vi "test TCX read (installed 71).vi"() -> ()   [LabVIEW 2011] (continued)
2\"><Watts>150</Watts></TPX></Extensions></Trackpoint><Trackpoint><Time>2008-03-03T23:14:53Z</Time><Position><LatitudeDegrees>35.869608</LatitudeDegrees><LongitudeDegrees>-78.914474</LongitudeDegrees></Position><AltitudeMeters>67.430</AltitudeMeters><DistanceMeters>16349.594</DistanceMeters><Cadence>80</Cadence><Extensions><TPX xmlns=\"http://www.garmin.com/xmlschemas/ActivityExtension/v2\"><Watts>150</Watts></TPX></Extensions></Trackpoint><Trackpoint><Time>2008-03-03T23:14:54Z</Time><Position><LatitudeDegrees>35.869697</LatitudeDegrees><LongitudeDegrees>-78.914429</LongitudeDegrees></Position><AltitudeMeters>66.949</AltitudeMeters><DistanceMeters>16360.299</DistanceMeters><Cadence>80</Cadence><Extensions><TPX xmlns=\"http://www.garmin.com/xmlschemas/ActivityExtension/v2\"><Watts>127</Watts></TPX></Extensions></Trackpoint><Trackpoint><Time>2008-03-03T23:14:55Z</Time><Position><LatitudeDegrees>35.869785</LatitudeDegrees><LongitudeDegrees>-78.914384</LongitudeDegrees></Position><AltitudeMeters>67.430</AltitudeMeters><DistanceMeters>16370.849</DistanceMeters><Cadence>80</Cadence><Extensions><TPX xmlns=\"http://www.garmin.com/xmlschemas/ActivityExtension/v2\"><Watts>124</Watts></TPX></Extensions></Trackpoint><Trackpoint><Time>2008-03-03T23:14:56Z</Time><Position><LatitudeDegrees>35.869873</LatitudeDegrees><LongitudeDegrees>-78.914337</LongitudeDegrees></Position><AltitudeMeters>67.430</AltitudeMeters><DistanceMeters>16381.465</DistanceMeters><Cadence>80</Cadence><Extensions><TPX xmlns=\"http://www.garmin.com/xmlschemas/ActivityExtension/v2\"><Watts>125</Watts></TPX></Extensions></Trackpoint><Trackpoint><Time>2008-03-03T23:14:57Z</Time><Position><LatitudeDegrees>35.869961</LatitudeDegrees><LongitudeDegrees>-78.914292</LongitudeDegrees></Position><AltitudeMeters>66.949</AltitudeMeters><DistanceMeters>16392.021</DistanceMeters><Cadence>81</Cadence><Extensions><TPX xmlns=\"http://www.garmin.com/xmlschemas/ActivityExtension/v2\"><Watts>138</Watts></TPX></Extensions></Trackpoint><Trackpoint><Time>2008-03-03T23:14:58Z</Time><Position><LatitudeDegrees>35.870049</LatitudeDegrees><LongitudeDegrees>-78.914246</LongitudeDegrees></Position><AltitudeMeters>66.468</AltitudeMeters><DistanceMeters>16402.668</DistanceMeters><Cadence>81</Cadence><Extensions><TPX xmlns=\"http://www.garmin.com/xmlschemas/ActivityExtension/v2\"><Watts>140</Watts></TPX></Extensions></Trackpoint><Trackpoint><Time>2008-03-03T23:14:59Z</Time><Position><LatitudeDegrees>35.870137</LatitudeDegrees><LongitudeDegrees>-78.914199</LongitudeDegrees></Position><AltitudeMeters>65.988</AltitudeMeters><DistanceMeters>16413.375</DistanceMeters><Cadence>81</Cadence><Extensions><TPX xmlns=\"http://www.garmin.com/xmlschemas/ActivityExtension/v2\"><Watts>126</Watts></TPX></Extensions></Trackpoint><Trackpoint><Time>2008-03-03T23:15:00Z</Time><Position><LatitudeDegrees>35.870228</LatitudeDegrees><LongitudeDegrees>-78.914151</LongitudeDegrees></Position><AltitudeMeters>65.507</AltitudeMeters><DistanceMeters>16424.277</DistanceMeters><Cadence>80</Cadence><Extensions><TPX xmlns=\"http://www.garmin.com/xmlschemas/ActivityExtension/v2\"><Watts>119</Watts></TPX></Extensions></Trackpoint><Trackpoint><Time>2008-03-03T23:15:01Z</Time><Position><LatitudeDegrees>35.870317</LatitudeDegrees><LongitudeDegrees>-78.914102</LongitudeDegrees></Position><AltitudeMeters>65.026</AltitudeMeters><DistanceMeters>16435.098</DistanceMeters><Cadence>78</Cadence><Extensions><TPX xmlns=\"http://www.garmin.com/xmlschemas/ActivityExtension/v2\"><Watts>109</Watts></TPX></Extensions></Trackpoint><Trackpoint><Time>2008-03-03T23:15:02Z</Time><Position><LatitudeDegrees>35.870407</LatitudeDegrees><LongitudeDegrees>-78.914053</LongitudeDegrees></Position><AltitudeMeters>65.026</AltitudeMeters><DistanceMeters>16446.086</DistanceMeters><Cadence>79</Cadence><Extensions><TPX xmlns=\"http://www.garmin.com/xmlschemas/ActivityExtension/v2\"><Watts>111</Watts></TPX></Extensions></Trackpoint><Trackpoint><Time>2008-03-03T23:15:03Z</Time><Position><LatitudeDegrees>35.870499</LatitudeDegrees><LongitudeDegrees>-78.914004</LongitudeDegrees></Position><AltitudeMeters>65.026</AltitudeMeters><DistanceMeters>16457.268</DistanceMeters><Cadence>80</Cadence><Extensions><TPX xmlns=\"http://www.garmin.com/xmlschemas/ActivityExtension/v2\"><Watts>116</Watts></TPX></Extensions></Trackpoint><Trackpoint><Time>2008-03-03T23:15:04Z</Time><Position><LatitudeDegrees>35.870594</LatitudeDegrees><LongitudeDegrees>-78.913954</LongitudeDegrees></Position><AltitudeMeters>64.065</AltitudeMeters><DistanceMeters>16468.787</DistanceMeters><Cadence>82</Cadence><Extensions><TPX xmlns=\"http://www.garmin.com/xmlschemas/ActivityExtension/v2\"><Watts>159</Watts></TPX></Extensions></Trackpoint><Trackpoint><Time>2008-03-03T23:15:05Z</Time><Position><LatitudeDegrees>35.870692</LatitudeDegrees><LongitudeDegrees>-78.913902</LongitudeDegrees></Position><AltitudeMeters>63.584</AltitudeMeters><DistanceMeters>16480.574</DistanceMeters><Cadence>84</Cadence><Extensions><TPX xmlns=\"http://www.garmin.com/xmlschemas/ActivityExtension/v2\"><Watts>189</Watts></TPX></Extensions></Trackpoint><Trackpoint><Time>2008-03-03T23:15:06Z</Time><Position><LatitudeDegrees>35.870793</LatitudeDegrees><LongitudeDegrees>-78.913849</LongitudeDegrees></Position><AltitudeMeters>63.584</AltitudeMeters><DistanceMeters>16492.729</DistanceMeters><Cadence>86</Cadence><Extensions><TPX xmlns=\"http://www.garmin.com/xmlschemas/ActivityExtension/v2\"><Watts>188</Watts></TPX></Extensions></Trackpoint><Trackpoint><Time>2008-03-03T23:15:07Z</Time><Position><LatitudeDegrees>35.870897</LatitudeDegrees><LongitudeDegrees>-78.913795</LongitudeDegrees></Position><AltitudeMeters>63.584</AltitudeMeters><DistanceMeters>16505.369</DistanceMeters><Cadence>88</Cadence><Extensions><TPX xmlns=\"http://www.garmin.com/xmlschemas/ActivityExtension/v2\"><Watts>169</Watts></TPX></Extensions></Trackpoint><Trackpoint><Time>2008-03-03T23:15:08Z</Time><Position><LatitudeDegrees>35.871002</LatitudeDegrees><LongitudeDegrees>-78.913740</LongitudeDegrees></Position><AltitudeMeters>63.104</AltitudeMeters><DistanceMeters>16518.016</DistanceMeters><Cadence>89</Cadence><Extensions><TPX xmlns=\"http://www.garmin.com/xmlschemas/ActivityExtension/v2\"><Watts>127</Watts></TPX></Extensions></Trackpoint><Trackpoint><Time>2008-03-03T23:15:09Z</Time><Position><LatitudeDegrees>35.871109</LatitudeDegrees><LongitudeDegrees>-78.913686</LongitudeDegrees></Position><AltitudeMeters>61.662</AltitudeMeters><DistanceMeters>16530.844</DistanceMeters><Cadence>92</Cadence><Extensions><TPX xmlns=\"http://www.garmin.com/xmlschemas/ActivityExtension/v2\"><Watts>98</Watts></TPX></Extensions></Trackpoint><Trackpoint><Time>2008-03-03T23:15:10Z</Time><Position><LatitudeDegrees>35.871217</LatitudeDegrees><LongitudeDegrees>-78.913629</LongitudeDegrees></Position><AltitudeMeters>62.142</AltitudeMeters><DistanceMeters>16543.873</DistanceMeters><Cadence>93</Cadence><Extensions><TPX xmlns=\"http://www.garmin.com/xmlschemas/ActivityExtension/v2\"><Watts>87</Watts></TPX></Extensions></Trackpoint><Trackpoint><Time>2008-03-03T23:15:11Z</Time><Position><LatitudeDegrees>35.871326</LatitudeDegrees><LongitudeDegrees>-78.913570</LongitudeDegrees></Position><AltitudeMeters>60.700</AltitudeMeters><DistanceMeters>16557.111</DistanceMeters><Cadence>88</Cadence><Extensions><TPX xmlns=\"http://www.garmin.com/xmlschemas/ActivityExtension/v2\"><Watts>91</Watts></TPX></Extensions></Trackpoint><Trackpoint><Time>2008-03-03T23:15:12Z</Time><Position><LatitudeDegrees>35.871438</LatitudeDegrees><LongitudeDegrees>-78.913510</LongitudeDegrees></Position><AltitudeMeters>60.700</AltitudeMeters><DistanceMeters>16570.666</DistanceMeters><Cadence>88</Cadence><Extensions><TPX xmlns=\"http://www.garmin.com/xmlschemas/ActivityExtension/v2\"><Watts>93</Watts></TPX></Extensions></Trackpoint><Trackpoint><Time>2008-03-03T23:15:13Z</Time><Position><LatitudeDegrees>35.871559</LatitudeDegrees><LongitudeDegrees>-78.913447</LongitudeDegrees></Position><AltitudeMeters>61.662</AltitudeMeters><DistanceMeters>16585.230</DistanceMeters><Cadence>90</Cadence><Extensions><TPX xmlns=\"http://www.garmin.com/xmlschemas/ActivityExtension/v2\"><Watts>100</Watts></TPX></Extensions></Trackpoint><Trackpoint><Time>2008-03-03T23:15:14Z</Time><Position><LatitudeDegrees>35.871675</LatitudeDegrees><LongitudeDegrees>-78.913392</LongitudeDegrees></Position><AltitudeMeters>59.739</AltitudeMeters><DistanceMeters>16599.100</DistanceMeters><Cadence>91</Cadence><Extensions><TPX xmlns=\"http://www.garmin.com/xmlschemas/ActivityExtension/v2\"><Watts>165</Watts></TPX></Extensions></Trackpoint><Trackpoint><Time>2008-03-03T23:15:15Z</Time><Position><LatitudeDegrees>35.871797</LatitudeDegrees><LongitudeDegrees>-78.913344</LongitudeDegrees></Position><AltitudeMeters>58.778</AltitudeMeters><DistanceMeters>16613.279</DistanceMeters><Cadence>91</Cadence><Extensions><TPX xmlns=\"http://www.garmin.com/xmlschemas/ActivityExtension/v2\"><Watts>165</Watts></TPX></Extensions></Trackpoint><Trackpoint><Time>2008-03-03T23:15:16Z</Time><Position><LatitudeDegrees>35.871917</LatitudeDegrees><LongitudeDegrees>-78.913298</LongitudeDegrees></Position><AltitudeMeters>58.778</AltitudeMeters><DistanceMeters>16627.301</DistanceMeters><Cadence>91</Cadence><Extensions><TPX xmlns=\"http://www.garmin.com/xmlschemas/ActivityExtension/v2\"><Watts>150</Watts></TPX></Extensions></Trackpoint><Trackpoint><Time>2008-03-03T23:15:17Z</Time><Position><LatitudeDegrees>35.872038</LatitudeDegrees><LongitudeDegrees>-78.913257</LongitudeDegrees></Position><AltitudeMeters>58.297</AltitudeMeters><DistanceMeters>16641.201</DistanceMeters><Cadence>91</Cadence><Extensions><TPX xmlns=\"http://www.garmin.com/xmlschemas/ActivityExtension/v2\"><Watts>129</Watts></TPX></Extensions></Trackpoint><Trackpoint><Time>2008-03-03T23:15:18Z</Time><Position><LatitudeDegrees>35.872160</LatitudeDegrees><LongitudeDegrees>-78.913222</LongitudeDegrees></Position><AltitudeMeters>57.817</AltitudeMeters><DistanceMeters>16655.086</DistanceMeters><Cadence>90</Cadence><Extensions><TPX xmlns=\"http://www.garmin.com/xmlschemas/ActivityExtension/v2\"><Watts>117</Watts></TPX></Extensions></Trackpoint><Trackpoint><Time>2008-03-03T23:15:19Z</Time><Position><LatitudeDegrees>35.872282</LatitudeDegrees><LongitudeDegrees>-78.913189</LongitudeDegrees></Position><AltitudeMeters>57.817</AltitudeMeters><DistanceMeters>16668.887</DistanceMeters><Cadence>88</Cadence><Extensions><TPX xmlns=\"http://www.garmin.com/xmlschemas/ActivityExtension/v2\"><Watts>97</Watts></TPX></Extensions></Trackpoint><Trackpoint><Time>2008-03-03T23:15:20Z</Time><Position><LatitudeDegrees>35.872398</LatitudeDegrees><LongitudeDegrees>-78.913161</LongitudeDegrees></Position><AltitudeMeters>58.778</AltitudeMeters><DistanceMeters>16682.076</DistanceMeters><Cadence>88</Cadence><Extensions><TPX xmlns=\"http://www.garmin.com/xmlschemas/ActivityExtension/v2\"><Watts>99</Watts></TPX></Extensions></Trackpoint><Trackpoint><Time>2008-03-03T23:15:21Z</Time><Position><LatitudeDegrees>35.872511</LatitudeDegrees><LongitudeDegrees>-78.913137</LongitudeDegrees></Position><AltitudeMeters>57.817</AltitudeMeters><DistanceMeters>16694.732</DistanceMeters><Cadence>83</Cadence><Extensions><TPX xmlns=\"http://www.garmin.com/xmlschemas/ActivityExtension/v2\"><Watts>83</Watts></TPX></Extensions></Trackpoint><Trackpoint><Time>2008-03-03T23:15:22Z</Time><Position><LatitudeDegrees>35.872627</LatitudeDegrees><LongitudeDegrees>-78.913118</LongitudeDegrees></Position><AltitudeMeters>58.297</AltitudeMeters><DistanceMeters>16707.732</DistanceMeters><Cadence>83</Cadence><Extensions><TPX xmlns=\"http://www.garmin.com/xmlschemas/ActivityExtension/v2\"><Watts>86</Watts></TPX></Extensions></Trackpoint><Trackpoint><Time>2008-03-03T23:15:23Z</Time><Position><LatitudeDegrees>35.872743</LatitudeDegrees><LongitudeDegrees>-78.913108</LongitudeDegrees></Position><AltitudeMeters>58.297</AltitudeMeters><DistanceMeters>16720.652</DistanceMeters><Cadence>82</Cadence><Extensions><TPX xmlns=\"http://www.garmin.com/xmlschemas/ActivityExtension/v2\"><Watts>108</Watts></TPX></Extensions></Trackpoint><Trackpoint><Time>2008-03-03T23:15:24Z</Time><Position><LatitudeDegrees>35.872857</LatitudeDegrees><LongitudeDegrees>-78.913113</LongitudeDegrees></Position><AltitudeMeters>58.297</AltitudeMeters><DistanceMeters>16733.250</DistanceMeters><Cadence>82</Cadence><Extensions><TPX xmlns=\"http://www.garmin.com/xmlschemas/ActivityExtension/v2\"><Watts>135</Watts></TPX></Extensions></Trackpoint><Trackpoint><Time>2008-03-03T23:15:25Z</Time><Position><LatitudeDegrees>35.872970</LatitudeDegrees><LongitudeDegrees>-78.913130</LongitudeDegrees></Position><AltitudeMeters>58.297</AltitudeMeters><DistanceMeters>16745.871</DistanceMeters><Cadence>82</Cadence><Extensions><TPX xmlns=\"http://www.garmin.com/xmlschemas/ActivityExtension/v2\"><Watts>133</Watts></TPX></Extensions></Trackpoint><Trackpoint><Time>2008-03-03T23:15:26Z</Time><Position><LatitudeDegrees>35.873082</LatitudeDegrees><LongitudeDegrees>-78.913155</LongitudeDegrees></Position><AltitudeMeters>58.778</AltitudeMeters><DistanceMeters>16758.455</DistanceMeters><Cadence>80</Cadence><Extensions><TPX xmlns=\"http://www.garmin.com/xmlschemas/ActivityExtension/v2\"><Watts>132</Watts></TPX></Extensions></Trackpoint><Trackpoint><Time>2008-03-03T23:15:27Z</Time><Position><LatitudeDegrees>35.873190</LatitudeDegrees><LongitudeDegrees>-78.913186</LongitudeDegrees></Position><AltitudeMeters>57.817</AltitudeMeters><DistanceMeters>16770.752</DistanceMeters><Cadence>80</Cadence><Extensions><TPX xmlns=\"http://www.garmin.com/xmlschemas/ActivityExtension/v2\"><Watts>131</Watts></TPX></Extensions></Trackpoint><Trackpoint><Time>2008-03-03T23:15:28Z</Time><Position><LatitudeDegrees>35.873294</LatitudeDegrees><LongitudeDegrees>-78.913223</LongitudeDegrees></Position><AltitudeMeters>58.297</AltitudeMeters><DistanceMeters>16782.869</DistanceMeters><Cadence>78</Cadence><Extensions><TPX xmlns=\"http://www.garmin.com/xmlschemas/ActivityExtension/v2\"><Watts>118</Watts></TPX></Extensions></Trackpoint><Trackpoint><Time>2008-03-03T23:15:29Z</Time><Position><LatitudeDegrees>35.873395</LatitudeDegrees><LongitudeDegrees>-78.913266</LongitudeDegrees></Position><AltitudeMeters>58.297</AltitudeMeters><DistanceMeters>16794.639</DistanceMeters><Cadence>75</Cadence><Extensions><TPX xmlns=\"http://www.garmin.com/xmlschemas/ActivityExtension/v2\"><Watts>120</Watts></TPX></Extensions></Trackpoint><Trackpoint><Time>2008-03-03T23:15:30Z</Time><Position><LatitudeDegrees>35.873490</LatitudeDegrees><LongitudeDegrees>-78.913316</LongitudeDegrees></Position><AltitudeMeters>57.336</AltitudeMeters><DistanceMeters>16806.027</DistanceMeters><Cadence>75</Cadence><Extensions><TPX xmlns=\"http://www.garmin.com/xmlschemas/ActivityExtension/v2\"><Watts>122</Watts></TPX></Extensions></Trackpoint><Trackpoint><Time>2008-03-03T23:15:31Z</Time><Position><LatitudeDegrees>35.873580</LatitudeDegrees><LongitudeDegrees>-78.913371</LongitudeDegrees></Position><AltitudeMeters>58.297</AltitudeMeters><DistanceMeters>16817.203</DistanceMeters><Cadence>73</Cadence><Extensions><TPX xmlns=\"http://www.garmin.com/xmlschemas/ActivityExtension/v2\"><Watts>130</Watts></TPX></Extensions></Trackpoint><Trackpoint><Time>2008-03-03T23:15:32Z</Time><Position><LatitudeDegrees>35.873667</LatitudeDegrees><LongitudeDegrees>-78.913428</LongitudeDegrees></Position><AltitudeMeters>57.817</AltitudeMeters><DistanceMeters>16828.195</DistanceMeters><Cadence>72</Cadence><Extensions><TPX xmlns=\"http://www.garmin.com/xmlschemas/ActivityExtension/v2\"><Watts>138</Watts></TPX></Extensions></Trackpoint><Trackpoint><Time>2008-03-03T23:15:33Z</Time><Position><LatitudeDegrees>35.873754</LatitudeDegrees><LongitudeDegrees>-78.913484</LongitudeDegrees></Position><AltitudeMeters>57.336</AltitudeMeters><DistanceMeters>16839.066</DistanceMeters><Cadence>71</Cadence><Extensions><TPX xmlns=\"http://www.garmin.com/xmlschemas/ActivityExtension/v2\"><Watts>136</Watts></TPX></Extensions></Trackpoint><Trackpoint><Time>2008-03-03T23:15:34Z</Time><Position><LatitudeDegrees>35.873838</LatitudeDegrees><LongitudeDegrees>-78.913541</LongitudeDegrees></Position><AltitudeMeters>57.336</AltitudeMeters><DistanceMeters>16849.713</DistanceMeters><Cadence>70</Cadence><Extensions><TPX xmlns=\"http://www.garmin.com/xmlschemas/ActivityExtension/v2\"><Watts>142</Watts></TPX></Extensions></Trackpoint><Trackpoint><Time>2008-03-03T23:15:35Z</Time><Position><LatitudeDegrees>35.873921</LatitudeDegrees><LongitudeDegrees>-78.913600</LongitudeDegrees></Position><AltitudeMeters>57.336</AltitudeMeters><DistanceMeters>16860.295</DistanceMeters><Cadence>69</Cadence><Extensions><TPX xmlns=\"http://www.garmin.com/xmlschemas/ActivityExtension/v2\"><Watts>153</Watts></TPX></Extensions></Trackpoint><Trackpoint><Time>2008-03-03T23:15:36Z</Time><Position><LatitudeDegrees>35.874004</LatitudeDegrees><LongitudeDegrees>-78.913657</LongitudeDegrees></Position><AltitudeMeters>56.855</AltitudeMeters><DistanceMeters>16870.801</DistanceMeters><Cadence>69</Cadence><Extensions><TPX xmlns=\"http://www.garmin.com/xmlschemas/ActivityExtension/v2\"><Watts>180</Watts></TPX></Extensions></Trackpoint><Trackpoint><Time>2008-03-03T23:15:37Z</Time><Position><LatitudeDegrees>35.874087</LatitudeDegrees><LongitudeDegrees>-78.913712</LongitudeDegrees></Position><AltitudeMeters>57.336</AltitudeMeters><DistanceMeters>16881.346</DistanceMeters><Cadence>69</Cadence><Extensions><TPX xmlns=\"http://www.garmin.com/xmlschemas/ActivityExtension/v2\"><Watts>179</Watts></TPX></Extensions></Trackpoint><Trackpoint><Time>2008-03-03T23:15:38Z</Time><Position><LatitudeDegrees>35.874169</LatitudeDegrees><LongitudeDegrees>-78.913768</LongitudeDegrees></Position><AltitudeMeters>57.336</AltitudeMeters><DistanceMeters>16891.715</DistanceMeters><Cadence>68</Cadence><Extensions><TPX xmlns=\"http://www.garmin.com/xmlschemas/ActivityExtension/v2\"><Watts>213</Watts></TPX></Extensions></Trackpoint><Trackpoint><Time>2008-03-03T23:15:39Z</Time><Position><LatitudeDegrees>35.874248</LatitudeDegrees><LongitudeDegrees>-78.913824</LongitudeDegrees></Position><AltitudeMeters>57.817</AltitudeMeters><DistanceMeters>16901.812</DistanceMeters><Cadence>71</Cadence><Extensions><TPX xmlns=\"http://www.garmin.com/xmlschemas/ActivityExtension/v2\"><Watts>213</Watts></TPX></Extensions></Trackpoint><Trackpoint><Time>2008-03-03T23:15:40Z</Time><Position><LatitudeDegrees>35.874326</LatitudeDegrees><LongitudeDegrees>-78.913878</LongitudeDegrees></Position><AltitudeMeters>57.817</AltitudeMeters><DistanceMeters>16911.746</DistanceMeters><Cadence>75</Cadence><Extensions><TPX xmlns=\"http://www.garmin.com/xmlschemas/ActivityExtension/v2\"><Watts>167</Watts></TPX></Extensions></Trackpoint><Trackpoint><Time>2008-03-03T23:15:41Z</Time><Position><LatitudeDegrees>35.874403</LatitudeDegrees><LongitudeDegrees>-78.913931</LongitudeDegrees></Position><AltitudeMeters>58.297</AltitudeMeters><DistanceMeters>16921.533</DistanceMeters><Cadence>74</Cadence><Extensions><TPX xmlns=\"http://www.garmin.com/xmlschemas/ActivityExtension/v2\"><Watts>165</Watts></TPX></Extensions></Trackpoint><Trackpoint><Time>2008-03-03T23:15:42Z</Time><Position><LatitudeDegrees>35.874479</LatitudeDegrees><LongitudeDegrees>-78.913982</LongitudeDegrees></Position><AltitudeMeters>58.297</AltitudeMeters><DistanceMeters>16931.109</DistanceMeters><Cadence>73</Cadence><Extensions><TPX xmlns=\"http://www.garmin.com/xmlschemas/ActivityExtension/v2\"><Watts>177</Watts></TPX></Extensions></Trackpoint><Trackpoint><Time>2008-03-03T23:15:43Z</Time><Position><LatitudeDegrees>35.874554</LatitudeDegrees><LongitudeDegrees>-78.914032</LongitudeDegrees></Position><AltitudeMeters>58.297</AltitudeMeters><DistanceMeters>16940.584</DistanceMeters><Cadence>72</Cadence><Extensions><TPX xmlns=\"http://www.garmin.com/xmlschemas/ActivityExtension/v2\"><Watts>199</Watts></TPX></Extensions></Trackpoint><Trackpoint><Time>2008-03-03T23:15:44Z</Time><Position><LatitudeDegrees>35.874628</LatitudeDegrees><LongitudeDegrees>-78.914082</LongitudeDegrees></Position><AltitudeMeters>58.778</AltitudeMeters><DistanceMeters>16949.957</DistanceMeters><Cadence>72</Cadence><Extensions><TPX xmlns=\"http://www.garmin.com/xmlschemas/ActivityExtension/v2\"><Watts>218</Watts></TPX></Extensions></Trackpoint><Trackpoint><Time>2008-03-03T23:15:45Z</Time><Position><LatitudeDegrees>35.874701</LatitudeDegrees><LongitudeDegrees>-78.914132</LongitudeDegrees></Position><AltitudeMeters>59.258</AltitudeMeters><DistanceMeters>16959.229</DistanceMeters><Cadence>72</Cadence><Extensions><TPX xmlns=\"http://www.garmin.com/xmlschemas/ActivityExtension/v2\"><Watts>219</Watts></TPX></Extensions></Trackpoint><Trackpoint><Time>2008-03-03T23:15:46Z</Time><Position><LatitudeDegrees>35.874774</LatitudeDegrees><LongitudeDegrees>-78.914181</LongitudeDegrees></Position><AltitudeMeters>59.258</AltitudeMeters><DistanceMeters>16968.434</DistanceMeters><Cadence>70</Cadence><Extensions><TPX xmlns=\"http://www.garmin.com/xmlschemas/ActivityExtension/v2\"><Watts>238</Watts></TPX></Extensions></Trackpoint><Trackpoint><Time>2008-03-03T23:15:47Z</Time><Position><LatitudeDegrees>35.874847</LatitudeDegrees><LongitudeDegrees>-78.914229</LongitudeDegrees></Position><AltitudeMeters>59.739</AltitudeMeters><DistanceMeters>16977.596</DistanceMeters><Cadence>70</Cadence><Extensions><TPX xmlns=\"http://www.garmin.com/xmlschemas/ActivityExtension/v2\"><Watts>245</Watts></TPX></Extensions></Trackpoint><Trackpoint><Time>2008-03-03T23:15:48Z</Time><Position><LatitudeDegrees>35.874918</LatitudeDegrees><LongitudeDegrees>-78.914277</LongitudeDegrees></Position><AltitudeMeters>59.739</AltitudeMeters><DistanceMeters>16986.635</DistanceMeters><Cadence>69</Cadence><Extensions><TPX xmlns=\"http://www.garmin.com/xmlschemas/ActivityExtension/v2\"><Watts>231</Watts></TPX></Extensions></Trackpoint><Trackpoint><Time>2008-03-03T23:15:49Z</Time><Position><LatitudeDegrees>35.874990</LatitudeDegrees><LongitudeDegrees>-78.914324</LongitudeDegrees></Position><AltitudeMeters>59.739</AltitudeMeters><DistanceMeters>16995.648</DistanceMeters><Cadence>69</Cadence><Extensions><TPX xmlns=\"http://www.garmin.com/xmlschemas/ActivityExtension/v2\"><Watts>219</Watts></TPX></Extensions></Trackpoint><Trackpoint><Time>2008-03-03T23:15:50Z</Time><Position><LatitudeDegrees>35.875060</LatitudeDegrees><LongitudeDegrees>-78.914373</LongitudeDegrees></Position><AltitudeMeters>59.739</AltitudeMeters><DistanceMeters>17004.566</DistanceMeters><Cadence>68</Cadence><Extensions><TPX xmlns=\"http://www.garmin.com/xmlschemas/ActivityExtension/v2\"><Watts>201</Watts></TPX></Extensions></Trackpoint><Trackpoint><Time>2008-03-03T23:15:51Z</Time><Position><LatitudeDegrees>35.875131</LatitudeDegrees><LongitudeDegrees>-78.914421</LongitudeDegrees></Position><AltitudeMeters>59.258</AltitudeMeters><DistanceMeters>17013.584</DistanceMeters><Cadence>68</Cadence><Extensions><TPX xmlns=\"http://www.garmin.com/xmlschemas/ActivityExtension/v2\"><Watts>204</Watts></TPX></Extensions></Trackpoint><Trackpoint><Time>2008-03-03T23:15:52Z</Time><Position><LatitudeDegrees>35.875200</LatitudeDegrees><LongitudeDegrees>-78.914470</LongitudeDegrees></Position><AltitudeMeters>59.258</AltitudeMeters><DistanceMeters>17022.492</DistanceMeters><Cadence>68</Cadence><Extensions><TPX xmlns=\"http://www.garmin.com/xmlschemas/ActivityExtension/v2\"><Watts>202</Watts></TPX></Extensions></Trackpoint><Trackpoint><Time>2008-03-03T23:15:53Z</Time><Position><LatitudeDegrees>35.875270</LatitudeDegrees><LongitudeDegrees>-78.914519</LongitudeDegrees></Position><AltitudeMeters>59.258</AltitudeMeters><DistanceMeters>17031.344</DistanceMeters><Cadence>68</Cadence><Extensions><TPX xmlns=\"http://www.garmin.com/xmlschemas/ActivityExtension/v2\"><Watts>189</Watts></TPX></Extensions></Trackpoint><Trackpoint><Time>2008-03-03T23:15:54Z</Time><Position><LatitudeDegrees>35.875341</LatitudeDegrees><LongitudeDegrees>-78.914566</LongitudeDegrees></Position><AltitudeMeters>58.778</AltitudeMeters><DistanceMeters>17040.268</DistanceMeters><Cadence>68</Cadence><Extensions><TPX xmlns=\"http://www.garmin.com/xmlschemas/ActivityExtension/v2\"><Watts>166</Watts></TPX></Extensions></Trackpoint><Trackpoint><Time>2008-03-03T23:15:55Z</Time><Position><LatitudeDegrees>35.875412</LatitudeDegrees><LongitudeDegrees>-78.914612</LongitudeDegrees></Position><AltitudeMeters>59.739</AltitudeMeters><DistanceMeters>17049.166</DistanceMeters><Cadence>68</Cadence><Extensions><TPX xmlns=\"http://www.garmin.com/xmlschemas/ActivityExtension/v2\"><Watts>168</Watts></TPX></Extensions></Trackpoint><Trackpoint><Time>2008-03-03T23:15:56Z</Time><Position><LatitudeDegrees>35.875483</LatitudeDegrees><LongitudeDegrees>-78.914654</LongitudeDegrees></Position><AltitudeMeters>59.258</AltitudeMeters><DistanceMeters>17057.984</DistanceMeters><Cadence>67</Cadence><Extensions><TPX xmlns=\"http://www.garmin.com/xmlschemas/ActivityExtension/v2\"><Watts>127</Watts></TPX></Extensions></Trackpoint><Trackpoint><Time>2008-03-03T23:15:57Z</Time><Position><LatitudeDegrees>35.875555</LatitudeDegrees><LongitudeDegrees>-78.914693</LongitudeDegrees></Position><AltitudeMeters>59.258</AltitudeMeters><DistanceMeters>17066.721</DistanceMeters><Cadence>67</Cadence><Extensions><TPX xmlns=\"http://www.garmin.com/xmlschemas/ActivityExtension/v2\"><Watts>118</Watts></TPX></Extensions></Trackpoint><Trackpoint><Time>2008-03-03T23:15:58Z</Time><Position><LatitudeDegrees>35.875628</LatitudeDegrees><LongitudeDegrees>-78.914729</LongitudeDegrees></Position><AltitudeMeters>59.739</AltitudeMeters><DistanceMeters>17075.404</DistanceMeters><Cadence>67</Cadence><Extensions><TPX xmlns=\"http://www.garmin.com/xmlschemas/ActivityExtension/v2\"><Watts>116</Watts></TPX></Extensions></Trackpoint><Trackpoint><Time>2008-03-03T23:15:59Z</Time><Position><LatitudeDegrees>35.875701</LatitudeDegrees><LongitudeDegrees>-78.914762</LongitudeDegrees></Position><AltitudeMeters>59.739</AltitudeMeters><DistanceMeters>17084.074</DistanceMeters><Cadence>66</Cadence><Extensions><TPX xmlns=\"http://www.garmin.com/xmlschemas/ActivityExtension/v2\"><Watts>124</Watts></TPX></Extensions></Trackpoint><Trackpoint><Time>2008-03-03T23:16:00Z</Time><Position><LatitudeDegrees>35.875773</LatitudeDegrees><LongitudeDegrees>-78.914796</LongitudeDegrees></Position><AltitudeMeters>60.700</AltitudeMeters><DistanceMeters>17092.635</DistanceMeters><Cadence>66</Cadence><Extensions><TPX xmlns=\"http://www.garmin.com/xmlschemas/ActivityExtension/v2\"><Watts>124</Watts></TPX></Extensions></Trackpoint><Trackpoint><Time>2008-03-03T23:16:01Z</Time><Position><LatitudeDegrees>35.875841</LatitudeDegrees><LongitudeDegrees>-78.914838</LongitudeDegrees></Position><AltitudeMeters>60.220</AltitudeMeters><DistanceMeters>17107.891</DistanceMeters><Cadence>65</Cadence><Extensions><TPX xmlns=\"http://www.garmin.com/xmlschemas/ActivityExtension/v2\"><Watts>69</Watts></TPX></Extensions></Trackpoint><Trackpoint><Time>2008-03-03T23:16:03Z</Time><Position><LatitudeDegrees>35.875934</LatitudeDegrees><LongitudeDegrees>-78.914975</LongitudeDegrees></Position><AltitudeMeters>59.739</AltitudeMeters><DistanceMeters>17120.564</DistanceMeters><Cadence>66</Cadence><Extensions><TPX xmlns=\"http://www.garmin.com/xmlschemas/ActivityExtension/v2\"><Watts>71</Watts></TPX></Extensions></Trackpoint><Trackpoint><Time>2008-03-03T23:16:04Z</Time><Position><LatitudeDegrees>35.875950</LatitudeDegrees><LongitudeDegrees>-78.915067</LongitudeDegrees></Position><AltitudeMeters>59.739</AltitudeMeters><DistanceMeters>17126.143</DistanceMeters><Cadence>66</Cadence><Extensions><TPX xmlns=\"http://www.garmin.com/xmlschemas/ActivityExtension/v2\"><Watts>168</Watts></TPX></Extensions></Trackpoint><Trackpoint><Time>2008-03-03T23:16:05Z</Time><Position><LatitudeDegrees>35.875952</LatitudeDegrees><LongitudeDegrees>-78.915164</LongitudeDegrees></Position><AltitudeMeters>59.739</AltitudeMeters><DistanceMeters>17134.875</DistanceMeters><Cadence>66</Cadence><Extensions><TPX xmlns=\"http://www.garmin.com/xmlschemas/ActivityExtension/v2\"><Watts>109</Watts></TPX></Extensions></Trackpoint><Trackpoint><Time>2008-03-03T23:16:06Z</Time><Position><LatitudeDegrees>35.875946</LatitudeDegrees><LongitudeDegrees>-78.915262</LongitudeDegrees></Position><AltitudeMeters>60.220</AltitudeMeters><DistanceMeters>17143.760</DistanceMeters><Cadence>67</Cadence><Extensions><TPX xmlns=\"http://www.garmin.com/xmlschemas/ActivityExtension/v2\"><Watts>120</Watts></TPX></Extensions></Trackpoint><Trackpoint><Time>2008-03-03T23:16:07Z</Time><Position><LatitudeDegrees>35.875939</LatitudeDegrees><LongitudeDegrees>-78.915361</LongitudeDegrees></Position><AltitudeMeters>59.739</AltitudeMeters><DistanceMeters>17152.768</DistanceMeters><Cadence>67</Cadence><Extensions><TPX xmlns=\"http://www.garmin.com/xmlschemas/ActivityExtension/v2\"><Watts>120</Watts></TPX></Extensions></Trackpoint><Trackpoint><Time>2008-03-03T23:16:08Z</Time><Position><LatitudeDegrees>35.875932</LatitudeDegrees><LongitudeDegrees>-78.915461</LongitudeDegrees></Position><AltitudeMeters>59.739</AltitudeMeters><DistanceMeters>17161.752</DistanceMeters><Cadence>68</Cadence><Extensions><TPX xmlns=\"http://www.garmin.com/xmlschemas/ActivityExtension/v2\"><Watts>160</Watts></TPX></Extensions></Trackpoint><Trackpoint><Time>2008-03-03T23:16:09Z</Time><Position><LatitudeDegrees>35.875925</LatitudeDegrees><LongitudeDegrees>-78.915561</LongitudeDegrees></Position><AltitudeMeters>59.739</AltitudeMeters><DistanceMeters>17170.854</DistanceMeters><Cadence>69</Cadence><Extensions><TPX xmlns=\"http://www.garmin.com/xmlschemas/ActivityExtension/v2\"><Watts>166</Watts></TPX></Extensions></Trackpoint><Trackpoint><Time>2008-03-03T23:16:10Z</Time><Position><LatitudeDegrees>35.875918</LatitudeDegrees><LongitudeDegrees>-78.915662</LongitudeDegrees></Position><AltitudeMeters>60.220</AltitudeMeters><DistanceMeters>17179.959</DistanceMeters><Cadence>69</Cadence><Extensions><TPX xmlns=\"http://www.garmin.com/xmlschemas/ActivityExtension/v2\"><Watts>155</Watts></TPX></Extensions></Trackpoint><Trackpoint><Time>2008-03-03T23:16:11Z</Time><Position><LatitudeDegrees>35.875910</LatitudeDegrees><LongitudeDegrees>-78.915762</LongitudeDegrees></Position><AltitudeMeters>59.739</AltitudeMeters><DistanceMeters>17189.072</DistanceMeters><Cadence>70</Cadence><Extensions><TPX xmlns=\"http://www.garmin.com/xmlschemas/ActivityExtension/v2\"><Watts>146</Watts></TPX></Extensions></Trackpoint><Trackpoint><Time>2008-03-03T23:16:12Z</Time><Position><LatitudeDegrees>35.875901</LatitudeDegrees><LongitudeDegrees>-78.915863</LongitudeDegrees></Position><AltitudeMeters>60.220</AltitudeMeters><DistanceMeters>17198.279</DistanceMeters><Cadence>70</Cadence><Extensions><TPX xmlns=\"http://www.garmin.com/xmlschemas/ActivityExtension/v2\"><Watts>138</Watts></TPX></Extensions></Trackpoint><Trackpoint><Time>2008-03-03T23:16:13Z</Time><Position><LatitudeDegrees>35.875891</LatitudeDegrees><LongitudeDegrees>-78.915965</LongitudeDegrees></Position><AltitudeMeters>60.220</AltitudeMeters><DistanceMeters>17207.531</DistanceMeters><Cadence>70</Cadence><Extensions><TPX xmlns=\"http://www.garmin.com/xmlschemas/ActivityExtension/v2\"><Watts>139</Watts></TPX></Extensions></Trackpoint><Trackpoint><Time>2008-03-03T23:16:14Z</Time><Position><LatitudeDegrees>35.875883</LatitudeDegrees><LongitudeDegrees>-78.916066</LongitudeDegrees></Position><AltitudeMeters>60.220</AltitudeMeters><DistanceMeters>17216.752</DistanceMeters><Cadence>70</Cadence><Extensions><TPX xmlns=\"http://www.garmin.com/xmlschemas/ActivityExtension/v2\"><Watts>138</Watts></TPX></Extensions></Trackpoint><Trackpoint><Time>2008-03-03T23:16:15Z</Time><Position><LatitudeDegrees>35.875875</LatitudeDegrees><LongitudeDegrees>-78.916169</LongitudeDegrees></Position><AltitudeMeters>59.739</AltitudeMeters><DistanceMeters>17226.062</DistanceMeters><Cadence>70</Cadence><Extensions><TPX xmlns=\"http://www.garmin.com/xmlschemas/ActivityExtension/v2\"><Watts>138</Watts></TPX></Extensions></Trackpoint><Trackpoint><Time>2008-03-03T23:16:16Z</Time><Position><LatitudeDegrees>35.875865</LatitudeDegrees><LongitudeDegrees>-78.916272</LongitudeDegrees></Position><AltitudeMeters>59.739</AltitudeMeters><DistanceMeters>17235.381</DistanceMeters><Cadence>71</Cadence><Extensions><TPX xmlns=\"http://www.garmin.com/xmlschemas/ActivityExtension/v2\"><Watts>137</Watts></TPX></Extensions></Trackpoint><Trackpoint><Time>2008-03-03T23:16:17Z</Time><Position><LatitudeDegrees>35.875857</LatitudeDegrees><LongitudeDegrees>-78.916375</LongitudeDegrees></Position><AltitudeMeters>59.258</AltitudeMeters><DistanceMeters>17244.721</DistanceMeters><Cadence>71</Cadence><Extensions><TPX xmlns=\"http://www.garmin.com/xmlschemas/ActivityExtension/v2\"><Watts>113</Watts></TPX></Extensions></Trackpoint><Trackpoint><Time>2008-03-03T23:16:18Z</Time><Position><LatitudeDegrees>35.875851</LatitudeDegrees><LongitudeDegrees>-78.916477</LongitudeDegrees></Position><AltitudeMeters>59.258</AltitudeMeters><DistanceMeters>17253.967</DistanceMeters><Cadence>71</Cadence><Extensions><TPX xmlns=\"http://www.garmin.com/xmlschemas/ActivityExtension/v2\"><Watts>103</Watts></TPX></Extensions></Trackpoint><Trackpoint><Time>2008-03-03T23:16:19Z</Time><Position><LatitudeDegrees>35.875842</LatitudeDegrees><LongitudeDegrees>-78.916581</LongitudeDegrees></Position><AltitudeMeters>59.258</AltitudeMeters><DistanceMeters>17263.408</DistanceMeters><Cadence>71</Cadence><Extensions><TPX xmlns=\"http://www.garmin.com/xmlschemas/ActivityExtension/v2\"><Watts>98</Watts></TPX></Extensions></Trackpoint><Trackpoint><Time>2008-03-03T23:16:20Z</Time><Position><LatitudeDegrees>35.875832</LatitudeDegrees><LongitudeDegrees>-78.916684</LongitudeDegrees></Position><AltitudeMeters>59.258</AltitudeMeters><DistanceMeters>17272.740</DistanceMeters><Cadence>72</Cadence><Extensions><TPX xmlns=\"http://www.garmin.com/xmlschemas/ActivityExtension/v2\"><Watts>100</Watts></TPX></Extensions></Trackpoint><Trackpoint><Time>2008-03-03T23:16:21Z</Time><Position><LatitudeDegrees>35.875823</LatitudeDegrees><LongitudeDegrees>-78.916787</LongitudeDegrees></Position><AltitudeMeters>59.258</AltitudeMeters><DistanceMeters>17282.199</DistanceMeters><Cadence>72</Cadence><Extensions><TPX xmlns=\"http://www.garmin.com/xmlschemas/ActivityExtension/v2\"><Watts>99</Watts></TPX></Extensions></Trackpoint><Trackpoint><Time>2008-03-03T23:16:22Z</Time><Position><LatitudeDegrees>35.875816</LatitudeDegrees><LongitudeDegrees>-78.916892</LongitudeDegrees></Position><AltitudeMeters>59.258</AltitudeMeters><DistanceMeters>17291.707</DistanceMeters><Cadence>73</Cadence><Extensions><TPX xmlns=\"http://www.garmin.com/xmlschemas/ActivityExtension/v2\"><Watts>104</Watts></TPX></Extensions></Trackpoint><Trackpoint><Time>2008-03-03T23:16:23Z</Time><Position><LatitudeDegrees>35.875808</LatitudeDegrees><LongitudeDegrees>-78.916998</LongitudeDegrees></Position><AltitudeMeters>59.258</AltitudeMeters><DistanceMeters>17301.322</DistanceMeters><Cadence>73</Cadence><Extensions><TPX xmlns=\"http://www.garmin.com/xmlschemas/ActivityExtension/v2\"><Watts>147</Watts></TPX></Extensions></Trackpoint><Trackpoint><Time>2008-03-03T23:16:24Z</Time><Position><LatitudeDegrees>35.875800</LatitudeDegrees><LongitudeDegrees>-78.917106</LongitudeDegrees></Position><AltitudeMeters>58.778</AltitudeMeters><DistanceMeters>17311.053</DistanceMeters><Cadence>74</Cadence><Extensions><TPX xmlns=\"http://www.garmin.com/xmlschemas/ActivityExtension/v2\"><Watts>180</Watts></TPX></Extensions></Trackpoint><Trackpoint><Time>2008-03-03T23:16:25Z</Time><Position><LatitudeDegrees>35.875788</LatitudeDegrees><LongitudeDegrees>-78.917214</LongitudeDegrees></Position><AltitudeMeters>58.778</AltitudeMeters><DistanceMeters>17320.893</DistanceMeters><Cadence>75</Cadence><Extensions><TPX xmlns=\"http://www.garmin.com/xmlschemas/ActivityExtension/v2\"><Watts>183</Watts></TPX></Extensions></Trackpoint><Trackpoint><Time>2008-03-03T23:16:26Z</Time><Position><LatitudeDegrees>35.875777</LatitudeDegrees><LongitudeDegrees>-78.917321</LongitudeDegrees></Position><AltitudeMeters>58.778</AltitudeMeters><DistanceMeters>17330.668</DistanceMeters><Cadence>75</Cadence><Extensions><TPX xmlns=\"http://www.garmin.com/xmlschemas/ActivityExtension/v2\"><Watts>185</Watts></TPX></Extensions></Trackpoint><Trackpoint><Time>2008-03-03T23:16:27Z</Time><Position><LatitudeDegrees>35.875763</LatitudeDegrees><LongitudeDegrees>-78.917430</LongitudeDegrees></Position><AltitudeMeters>58.778</AltitudeMeters><DistanceMeters>17340.646</DistanceMeters><Cadence>74</Cadence><Extensions><TPX xmlns=\"http://www.garmin.com/xmlschemas/ActivityExtension/v2\"><Watts>167</Watts></TPX></Extensions></Trackpoint><Trackpoint><Time>2008-03-03T23:16:28Z</Time><Position><LatitudeDegrees>35.875747</LatitudeDegrees><LongitudeDegrees>-78.917539</LongitudeDegrees></Position><AltitudeMeters>59.258</AltitudeMeters><DistanceMeters>17350.613</DistanceMeters><Cadence>74</Cadence><Extensions><TPX xmlns=\"http://www.garmin.com/xmlschemas/ActivityExtension/v2\"><Watts>154</Watts></TPX></Extensions></Trackpoint><Trackpoint><Time>2008-03-03T23:16:29Z</Time><Position><LatitudeDegrees>35.875736</LatitudeDegrees><LongitudeDegrees>-78.917646</LongitudeDegrees></Position><AltitudeMeters>59.258</AltitudeMeters><DistanceMeters>17360.293</DistanceMeters><Cadence>73</Cadence><Extensions><TPX xmlns=\"http://www.garmin.com/xmlschemas/ActivityExtension/v2\"><Watts>155</Watts></TPX></Extensions></Trackpoint><Trackpoint><Time>2008-03-03T23:16:30Z</Time><Position><LatitudeDegrees>35.875725</LatitudeDegrees><LongitudeDegrees>-78.917751</LongitudeDegrees></Position><AltitudeMeters>59.258</AltitudeMeters><DistanceMeters>17369.906</DistanceMeters><Cadence>71</Cadence><Extensions><TPX xmlns=\"http://www.garmin.com/xmlschemas/ActivityExtension/v2\"><Watts>156</Watts></TPX></Extensions></Trackpoint><Trackpoint><Time>2008-03-03T23:16:31Z</Time><Position><LatitudeDegrees>35.875715</LatitudeDegrees><LongitudeDegrees>-78.917855</LongitudeDegrees></Position><AltitudeMeters>59.258</AltitudeMeters><DistanceMeters>17379.350</DistanceMeters><Cadence>74</Cadence><Extensions><TPX xmlns=\"http://www.garmin.com/xmlschemas/ActivityExtension/v2\"><Watts>150</Watts></TPX></Extensions></Trackpoint><Trackpoint><Time>2008-03-03T23:16:32Z</Time><Position><LatitudeDegrees>35.875709</LatitudeDegrees><LongitudeDegrees>-78.917958</LongitudeDegrees></Position><AltitudeMeters>59.258</AltitudeMeters><DistanceMeters>17388.732</DistanceMeters><Cadence>84</Cadence><Extensions><TPX xmlns=\"http://www.garmin.com/xmlschemas/ActivityExtension/v2\"><Watts>148</Watts></TPX></Extensions></Trackpoint><Trackpoint><Time>2008-03-03T23:16:33Z</Time><Position><LatitudeDegrees>35.875701</LatitudeDegrees><LongitudeDegrees>-78.918060</LongitudeDegrees></Position><AltitudeMeters>59.258</AltitudeMeters><DistanceMeters>17397.910</DistanceMeters><Cadence>83</Cadence><Extensions><TPX xmlns=\"http://www.garmin.com/xmlschemas/ActivityExtension/v2\"><Watts>182</Watts></TPX></Extensions></Trackpoint><Trackpoint><Time>2008-03-03T23:16:34Z</Time><Position><LatitudeDegrees>35.875692</LatitudeDegrees><LongitudeDegrees>-78.918160</LongitudeDegrees></Position><AltitudeMeters>59.258</AltitudeMeters><DistanceMeters>17406.957</DistanceMeters><Cadence>83</Cadence><Extensions><TPX xmlns=\"http://www.garmin.com/xmlschemas/ActivityExtension/v2\"><Watts>181</Watts></TPX></Extensions></Trackpoint><Trackpoint><Time>2008-03-03T23:16:35Z</Time><Position><LatitudeDegrees>35.875682</LatitudeDegrees><LongitudeDegrees>-78.918260</LongitudeDegrees></Position><AltitudeMeters>60.220</AltitudeMeters><DistanceMeters>17416.070</DistanceMeters><Cadence>84</Cadence><Extensions><TPX xmlns=\"http://www.garmin.com/xmlschemas/ActivityExtension/v2\"><Watts>217</Watts></TPX></Extensions></Trackpoint><Trackpoint><Time>2008-03-03T23:16:36Z</Time><Position><LatitudeDegrees>35.875673</LatitudeDegrees><LongitudeDegrees>-78.918360</LongitudeDegrees></Position><AltitudeMeters>59.73
